vi "Reset Simulation.vi"(0 "reference in":refnum<class "Battery.lvclass">, 5 "Error In":errorcluster) -> (14 "reference out":refnum<class "Battery.lvclass">, 16 "simulation reset":bool, 19 "Error Out":errorcluster)   [LabVIEW 2023, in "Battery.lvclass"]
uses:
  Battery.lvclass
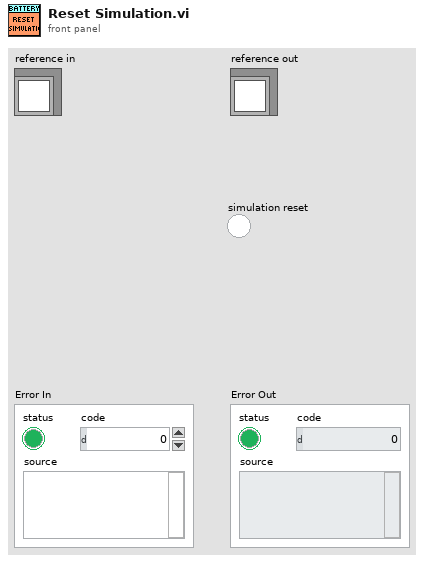
[diagram p1: front panel]
types:
  T1 = typedef "Battery.lvclass/ObjectAttributes.ctl" = cluster{"Python module":path, "Python Session":refnum<k35>, "PybammWrapper":refnum<k38>, "simulation loaded":bool, "simulation enabled":bool, "SOC OCV Curve":dbl[][], "Open Circuit Voltage (V)":dbl, "Terminal Voltage (V)":dbl, "State of Charge (%)":dbl, "# Cells in Series":u16, "# Cells in Parallel":u16, "Simulation Parameters":T2, "Power Module":refnum<class "PowerModuleInterface.lvclass">}
  T2 = typedef "Battery.lvclass/Simulation Parameters.ctl" = cluster{"num_rc_pairs":i32, "R0":dbl, "R1":dbl, "C1":dbl, "R2":dbl, "C2":dbl, " nominal_capacity_Ah":dbl, "upper_voltage_cutoff":dbl, "lower_voltage_cutoff":dbl}
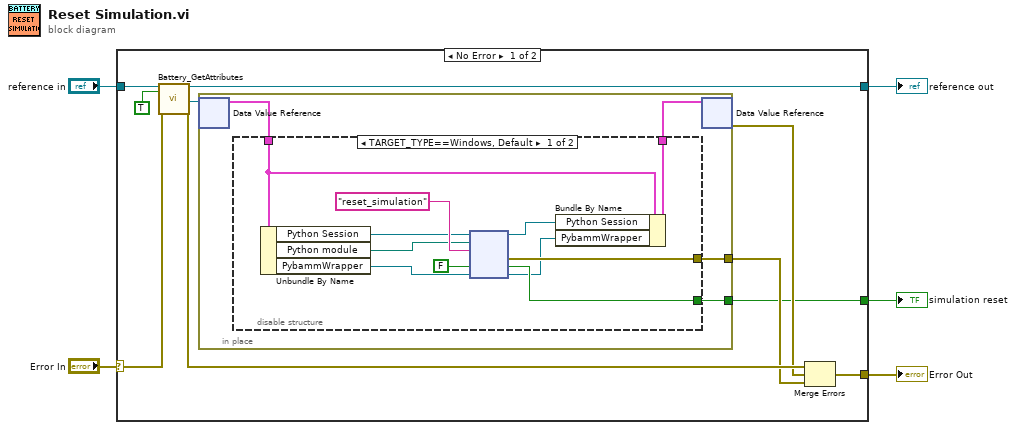
[diagram p0: block diagram]
diagram:
  n1 = case shown="No Error" "Error In" {
    selector: "Error In" -> [w14 w33]
    tunnel: [w12 w33] -> w4
    tunnel: [w13 w32] -> w2
    tunnel: "reference in" -> [w15 w32]
    tunnel: [w6 _] -> w1
    frame No Error {
      n2 = call "Battery_GetAttributes.vi"("reference in"=w15, "OnlyGetDvrReference(False)"=TRUE, "Error In"=w14) -> ("reference out"=w13:refnum<class "Battery.lvclass">, "DataRef"=w11:refnum<data-value>, "Error Out"=w9:errorcluster)  [unwired: 13 in, 1 out]
      n3 = in-place {
        in-place-border: [w19] -> w7
        in-place-border: [w18] -> w6
        n4 = in-place-dvr #1(w11) -> (w17:T1)  [unwired: 1 out]
        n5 = disable-structure shown="TARGET_TYPE==Windows, Default" {
          disable-tunnel: [w26 _] -> w19
          disable-tunnel: [w25 _] -> w18
          disable-tunnel: w17 -> [w24 w31]
          disable-tunnel: [w23 w31] -> w16
          frame condition #0 (active) {
            n6 = Unbundle By Name(w24) -> ("Python Session"=w28:refnum<k35>, "Python module"=w27:path, "PybammWrapper"=w29:refnum<k38>)
            n7 = node(w28, w27, "reset_simulation" ("function name"), FALSE, w29) -> (w21:refnum<k35>, w26:errorcluster, w25:bool, w22:refnum<k38>)  [unwired: 1 in, 2 out]
            n8 = Bundle By Name(cluster=w24, "Python Session"=w21, "PybammWrapper"=w22) -> (w23:T1)
          }
          frame condition #1 {
          }
        }
        n9 = in-place-dvr #1(w16) -> (w8:errorcluster)  [unwired: 1 out]
      }
      n10 = Merge Errors(w9, w8, w7) -> (w12:errorcluster)
    }
    frame Error {
    }
  }
  "Error Out" <- w4
  "reference out" <- w2
  "simulation reset" <- w1
